vi "Select Profiles.vi"(8 "error in (no error)":errorcluster) -> (0 "error out":errorcluster, 2 "Profile Out":string, 3 "LBCB  Location Out":T1)   [LabVIEW 2013]
uses:
  lib/Data Access Objects/Metadata/LBCB Location.ctl
  lib/Data Access Objects/Metadata/Persistant DAO Actions.ctl
panel:
  in  "Advanced":bool
  in  "Ok":bool
  in  "Clone":bool
  in  "Select Profile":i32(listbox)
  in  "OM  Location":T1
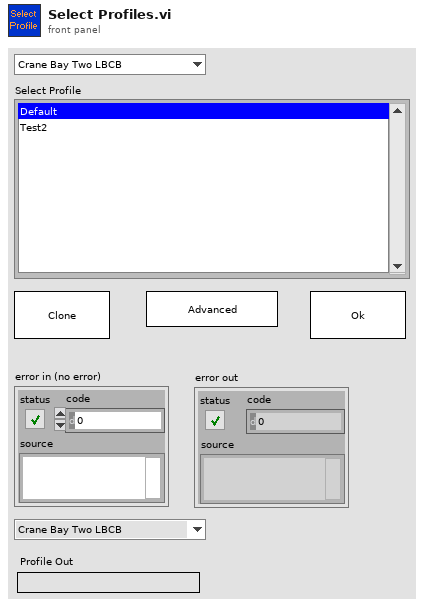
[diagram p1: front panel]
types:
  T1 = typedef "LBCB Location.ctl" = enum16{"Crane Bay Two LBCB", "Crane Bay One LBCB", "5th Scale Two LBCB", "5th Scale One LBCB", "Portable LBCB", "University of Houston LBCB"}
  T2 = typedef "Persistant DAO Actions.ctl" = enum16{"Init", "Get", "Set", "Load", "Save"}
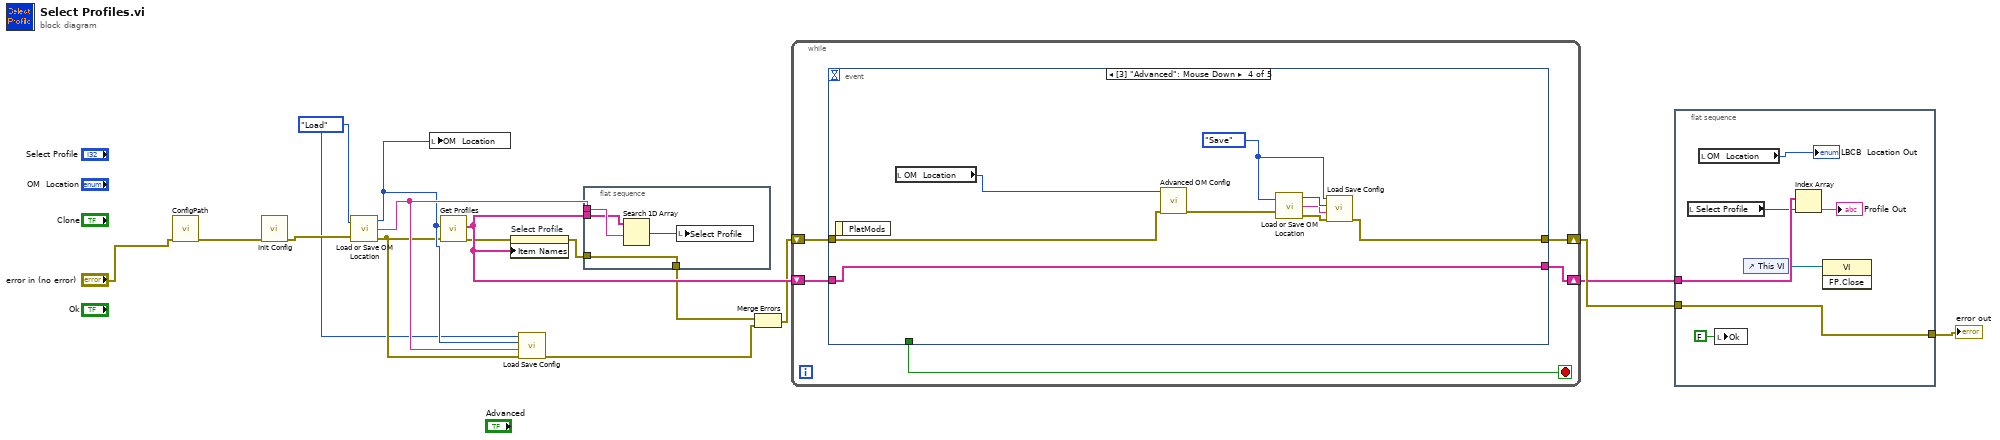
[diagram p0: block diagram]
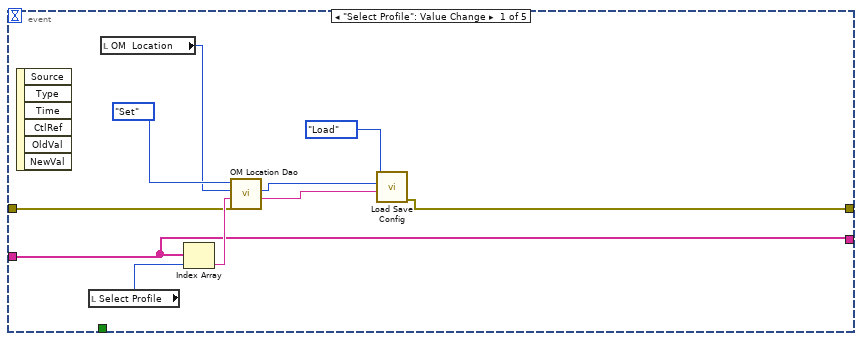
[diagram p2: hidden frame]
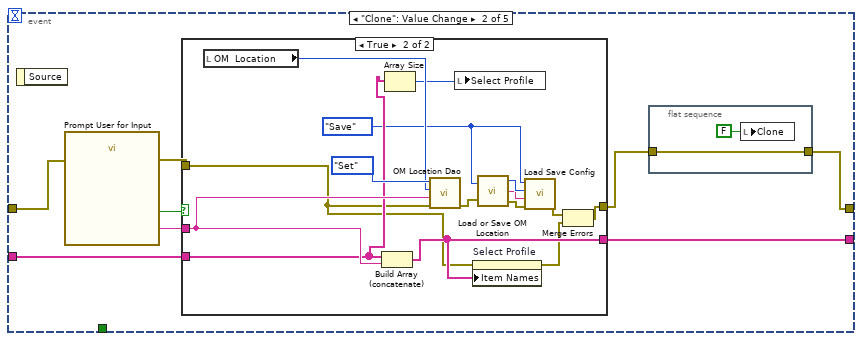
[diagram p3: hidden frame]
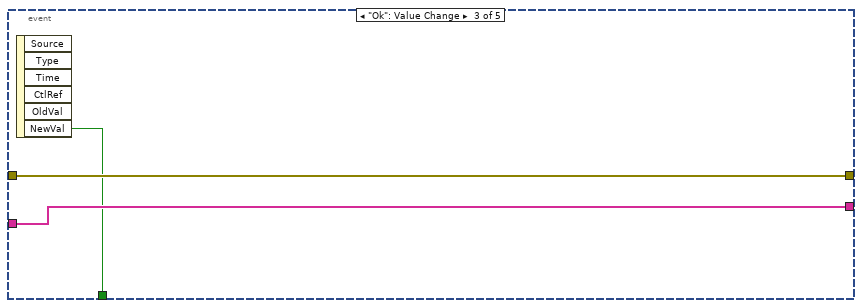
[diagram p5: hidden frame]
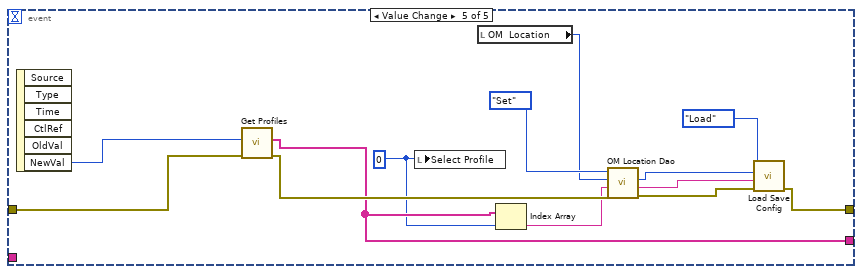
[diagram p6: hidden frame]
diagram:
  w1 = Persistant_DAO_Actions."Load" ("Action")
  n1 = call "ConfigPath.vi"("error in (no error)"="error in (no error)") -> ("error out"=w8:errorcluster)  [unwired: 8 in, 2 out]
  n2 = call "Init Config.vi"("error in (no error)"=w8) -> ("error out"=w7:errorcluster)  [unwired: 10 in]
  n3 = call "Load or Save OM Location.vi"("Action"=w1, "error in (no error)"=w7) -> ("LBCB  Location Out"=w5:T1, "Profile"=w6:string, "error out"=w2:errorcluster)
  n4 = local write "OM  Location"(w5) -> ()
  n5 = call "Get Profiles.vi"("error in"=w2, "OM  Location"=w5) -> ("error out"=w15:errorcluster, "folder names"=w16:string[])  [unwired: 8 in]
  n6 = property on="Select Profile" class="LstBox (strict)"(error in=w15, "Item Names"=w16) -> (error out=w14:errorcluster)  [unwired: 1 in, 1 out]
  n7 = call "Load Save Config.vi"("error in (no error)"=w2, "Profile"=w6, "OM  Location"=w5, "Actions"=w1) -> ("error out"=w3:errorcluster)  [unwired: 7 in]
  n8 = flat-sequence {
    tunnel: w6 -> [w20]
    tunnel: w16 -> [w18]
    tunnel: w14 -> [w17]
    tunnel: [w17] -> w13
    frame #0 {
      n9 = Search 1D Array(1D array=w18, element=w20) -> (index of element=w19:i32)  [unwired: 1 in]
      n10 = local write "Select Profile"(w19) -> ()
    }
  }
  n11 = Merge Errors(w13, w3) -> (w4:errorcluster)
  n12 = while {
    shift-right: [w23] -> w12
    shift-left: w4 -> [w24]
    shift-right: [w22] -> w10
    shift-left: w16 -> [w25]
    stop <- w21 stop-if-true
    n13 = event shown="[3] \"Advanced\": Mouse Down" {
      selector: _ -> [_ _ _ _ _]
      dyn-events: _ -> [_ _ _ _ _]
      timeout: _ -> [_ _ _ _ _]
      tunnel: w25 -> [w30 w39 w65 w73 _]
      tunnel: w24 -> [w31 w43 w64 w68 w87]
      tunnel: [w26 w36 w64 w67 w78] -> w23
      tunnel: [w30 w38 w65 w73 w77] -> w22
      tunnel: [_ _ w63 _ _] -> w21
      event "Select Profile": Value Change {
        n14 = event-data() -> ()  [unwired: 1 in, 6 out]
        n15 = local read "Select Profile"() -> (w33:i32)
        n16 = local read "OM  Location"() -> (w34:T1)
        n17 = Index Array(array=w30, index=w33) -> (element=w32:string)
        n18 = call "OM Location Dao.vi"("error in (no error)"=w31, "Profile In"=w32, "LBCB  Location In"=w34, "Actions"=Persistant_DAO_Actions."Set") -> ("Profile Out"=w27:string, "LBCB  Location Out"=w28:T1)  [unwired: 4 in, 2 out]
        n19 = call "Load Save Config.vi"("Profile"=w27, "OM  Location"=w28, "Actions"=Persistant_DAO_Actions."Load") -> ("error out"=w26:errorcluster)  [unwired: 8 in]
      }
      event "Clone": Value Change {
        n20 = event-data() -> ()  [unwired: 1 in, 1 out]
        n21 = call "Prompt User for Input"("error in (no error)"=w43) -> ("Profile Name"=w40:string, "OK"=w41:bool, "error out"=w42:errorcluster)  [unwired: 16 in]
        n22 = case shown="True" w41 {
          tunnel: w39 -> [w47 w57]
          tunnel: [w46 w49] -> w37
          tunnel: w42 -> [w46 w52]
          tunnel: w40 -> [_ w59]
          tunnel: [w47 w58] -> w38
          frame False {
          }
          frame True {
            w48 = Persistant_DAO_Actions."Save" ("Action")
            n23 = local read "OM  Location"() -> (w61:T1)
            n24 = Build Array (concatenate)(w57, w59) -> (w58:string[])
            n25 = Array Size(array=w57) -> (size(s)=w60:i32)
            n26 = call "OM Location Dao.vi"("error in (no error)"=w52, "Profile In"=w59, "LBCB  Location In"=w61, "Actions"=Persistant_DAO_Actions."Set") -> ("error out"=w53:errorcluster)  [unwired: 4 in, 3 out]
            n27 = local write "Select Profile"(w60) -> ()
            n28 = property on="Select Profile" class="LstBox (strict)"(error in=w52, "Item Names"=w58) -> (error out=w50:errorcluster)  [unwired: 1 in, 1 out]
            n29 = call "Load or Save OM Location.vi"("Action"=w48, "error in (no error)"=w53) -> ("LBCB  Location Out"=w56:T1, "Profile"=w55:string, "error out"=w54:errorcluster)
            n30 = call "Load Save Config.vi"("error in (no error)"=w54, "Profile"=w55, "OM  Location"=w56, "Actions"=w48) -> ("error out"=w51:errorcluster)  [unwired: 7 in]
            n31 = Merge Errors(w51, w50) -> (w49:errorcluster)
          }
        }
        n32 = flat-sequence {
          tunnel: w37 -> [w45]
          tunnel: [w45] -> w36
          frame #0 {
            n33 = local write "Clone"(FALSE ("Select")) -> ()
          }
        }
      }
      event "Ok": Value Change {
        n34 = event-data() -> ("NewVal"=w63:bool)  [unwired: 1 in, 5 out]
      }
      event "Advanced": Mouse Down {
        w66 = Persistant_DAO_Actions."Save" ("Action")
        n35 = event-data() -> ()  [unwired: 1 in, 1 out]
        n36 = local read "OM  Location"() -> (w74:T1)
        n37 = call "Advanced OM Config.vi"("error in (no error)"=w68, "OM  Location"=w74) -> ("error out"=w69:errorcluster)  [unwired: 9 in]
        n38 = call "Load or Save OM Location.vi"("Action"=w66, "error in (no error)"=w69) -> ("LBCB  Location Out"=w72:T1, "Profile"=w71:string, "error out"=w70:errorcluster)
        n39 = call "Load Save Config.vi"("error in (no error)"=w70, "Profile"=w71, "OM  Location"=w72, "Actions"=w66) -> ("error out"=w67:errorcluster)  [unwired: 7 in]
      }
      event Value Change {
        w76 = 0
        n40 = event-data() -> ("NewVal"=w86:T1)  [unwired: 1 in, 5 out]
        n41 = call "Get Profiles.vi"("error in"=w87, "OM  Location"=w86) -> ("error out"=w80:errorcluster, "folder names"=w77:string[])  [unwired: 8 in]
        n42 = local write "Select Profile"(w76) -> ()
        n43 = local read "OM  Location"() -> (w84:T1)
        n44 = Index Array(array=w77, index=w76) -> (element=w75:string)
        n45 = call "OM Location Dao.vi"("error in (no error)"=w80, "Profile In"=w75, "LBCB  Location In"=w84, "Actions"=Persistant_DAO_Actions."Set") -> ("error out"=w79:errorcluster, "Profile Out"=w81:string, "LBCB  Location Out"=w82:T1)  [unwired: 4 in, 1 out]
        n46 = call "Load Save Config.vi"("error in (no error)"=w79, "Profile"=w81, "OM  Location"=w82, "Actions"=Persistant_DAO_Actions."Load") -> ("error out"=w78:errorcluster)  [unwired: 7 in]
      }
    }
  }
  n47 = flat-sequence {
    tunnel: w12 -> [w93]
    tunnel: [w93] -> w11
    tunnel: w10 -> [w91]
    frame #0 {
      n48 = local read "Select Profile"() -> (w90:i32)
      n49 = local read "OM  Location"() -> (→"LBCB  Location Out":T1)
      n50 = local write "Ok"(FALSE ("Ok")) -> ()
      n51 = control-ref of="This VI"() -> (w88:refnum<vi>)
      n52 = Index Array(array=w91, index=w90) -> (element=→"Profile Out":string)
      n53 = invoke class="VI" method="FP.Close"(reference=w88) -> ()  [unwired: 2 in, 3 out]
    }
  }
  "error out" <- w11
